vi "Move Front Panel Objects.vi"(5 "Y_Buffer":u32=20, 7 "X_Buffer":u32=20, 8 "Error In":errorcluster, 11 "FP Data":T1) -> (0 "Error Out":errorcluster, 3 "FP Data":T1)   [LabVIEW 2020, in "LMH-Toolbox.lvlib" / "LMH-Front-Panel-Clean-Up.lvlib"]
uses:
  LMH-Front-Panel-Clean-Up.lvlib
  Type Defs/FP Data.ctl
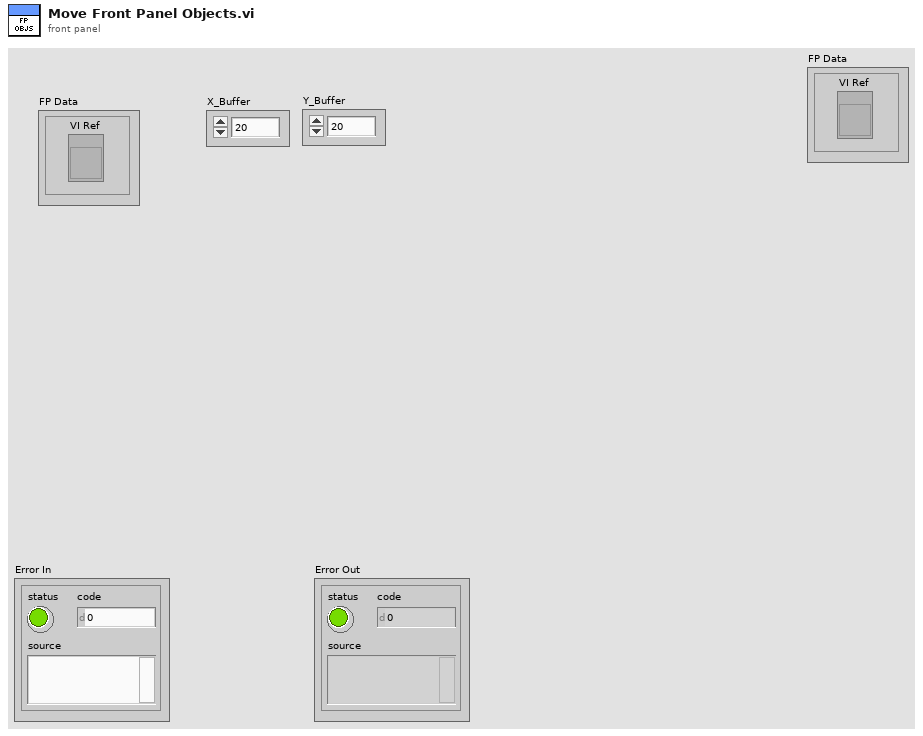
[diagram p1: front panel]
types:
  T1 = typedef "LMH-Toolbox.lvlib/LMH-Front-Panel-Clean-Up.lvlib/FP Data.ctl" = cluster{"VI Ref":refnum<vi>, "FP Objects":refnum<vi>[][], "FP Object Names":string[][], "Max Widths":u32[], "Max Heights":u32[]}
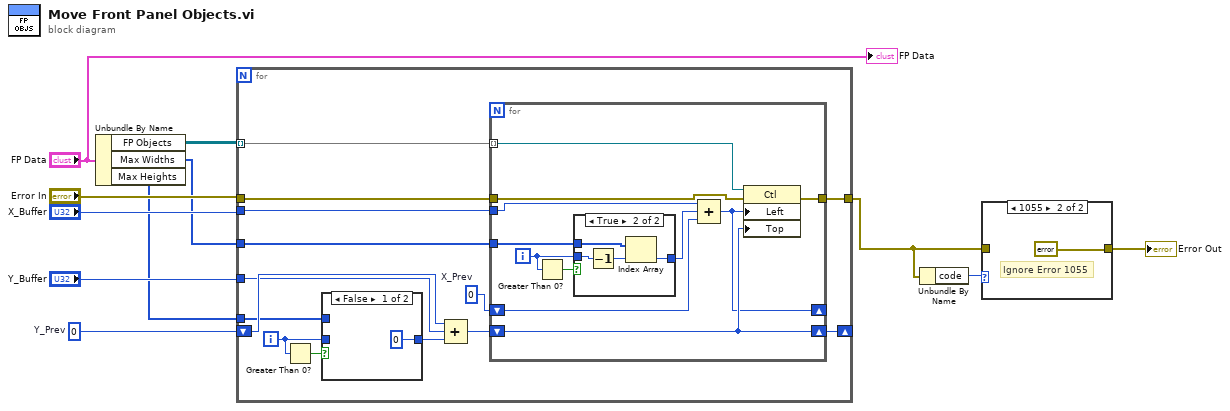
[diagram p0: block diagram]
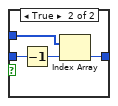
[diagram p3: hidden frame]
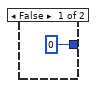
[diagram p4: hidden frame]
diagram:
  w9 = u32 0  # Y_Prev
  n1 = Unbundle By Name("FP Data") -> ("FP Objects"=w7:refnum<vi>[][], "Max Widths"=w6:u32[], "Max Heights"=w5:u32[])
  n2 = for {
    tunnel: w7 -> [w25] mode=indexing
    shift-right: [w24] -> _
    shift-left: w9 -> [w20]
    tunnel: "Error In" -> [w22]
    tunnel: [w21] -> w1
    tunnel: w5 -> [w19]
    tunnel: "Y_Buffer" -> [w15]
    tunnel: w6 -> [w14]
    tunnel: "X_Buffer" -> [w12]
    i -> [w17]
    w13 = u32 0  # X_Prev
    n3 = Greater Than 0?(x=w17) -> (x > 0?=w18:bool)
    n4 = case shown="False" w18 {
      tunnel: w19 -> [_ w30]
      tunnel: w17 -> [_ w28]
      tunnel: [u32 0 w27] -> w16
      frame False {
      }
      frame True {
        n5 = Decrement(x=w28) -> (x-1=w29:i32)
        n6 = Index Array(array=w30, index=w29) -> (element=w27:u32)
      }
    }
    n7 = Compound Arithmetic op=ADD(w20, w15, w16) -> (w23:u32)
    n8 = for {
      tunnel: w25 -> [w41] mode=indexing
      shift-right: [w38] -> w24
      shift-left: w23 -> [w38]
      tunnel: w22 -> [w40]
      tunnel: [w39] -> w21
      tunnel: w14 -> [w36]
      shift-right: [w32] -> _
      shift-left: w13 -> [w33]
      tunnel: w12 -> [w31]
      i -> [w35]
      n9 = Greater Than 0?(x=w35) -> (x > 0?=w37:bool)
      n10 = case shown="True" w37 {
        tunnel: w36 -> [_ w46]
        tunnel: [u32 0 w44] -> w34
        tunnel: w35 -> [_ w43]
        frame False {
        }
        frame True {
          n11 = Decrement(x=w43) -> (x-1=w45:i32)
          n12 = Index Array(array=w46, index=w45) -> (element=w44:u32)
        }
      }
      n13 = Compound Arithmetic op=ADD(w31, w34, w33) -> (w32:u32)
      n14 = property class="Ctl"(reference=w41, error in=w40, "Left"=w32, "Top"=w38) -> (error out=w39:errorcluster)  [unwired: 1 out]
    }
  }
  n15 = Unbundle By Name(w1) -> ("code"=w2:i32)
  n16 = case shown="1055" w2 {
    tunnel: [w47 errorcluster {"status"=FALSE, "code"=0, "source"=""} ("error out")] -> w3
    tunnel: w1 -> [w47 _]
    frame 0, Default {
    }
    frame 1055 {
      # "Ignore Error 1055"
    }
  }
  "Error Out" <- w3
  "FP Data" <- "FP Data"
